vi "HipEXO_SM_BioTorq.vi"(6 "Ext T":dbl, 9 "Trigger Ratio":dbl, 10 "Flex T":dbl, 11 "Hip Angle":dbl) -> (1 "GC Duration":u32, 2 "Extension":bool=TRUE, 3 "Flexion":bool=TRUE, 4 "Output Torque":dbl)   [LabVIEW 2018]
uses:
  <vilib>/functionblocks/Edge Detection/One Shot Rising with Input/One Shot Rising with Input.vi
  <vilib>/functionblocks/FB Core/FB Core.xnode
  <vilib>/functionblocks/NI_FunctionBlock Libraries.lvlib
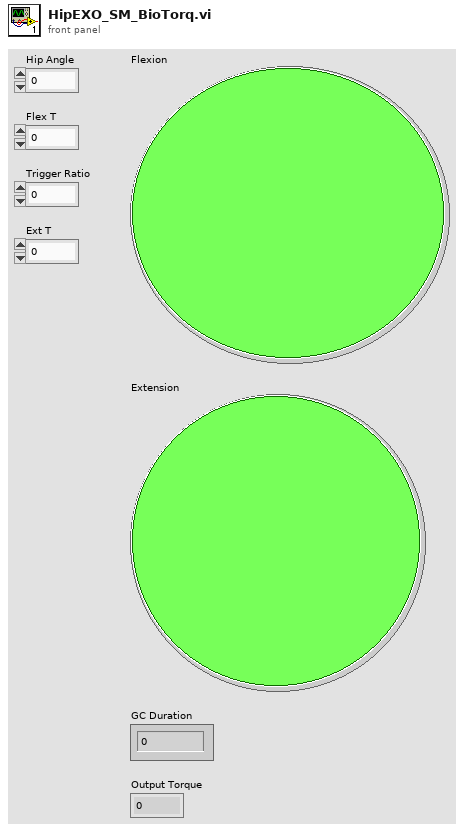
[diagram p1: front panel]
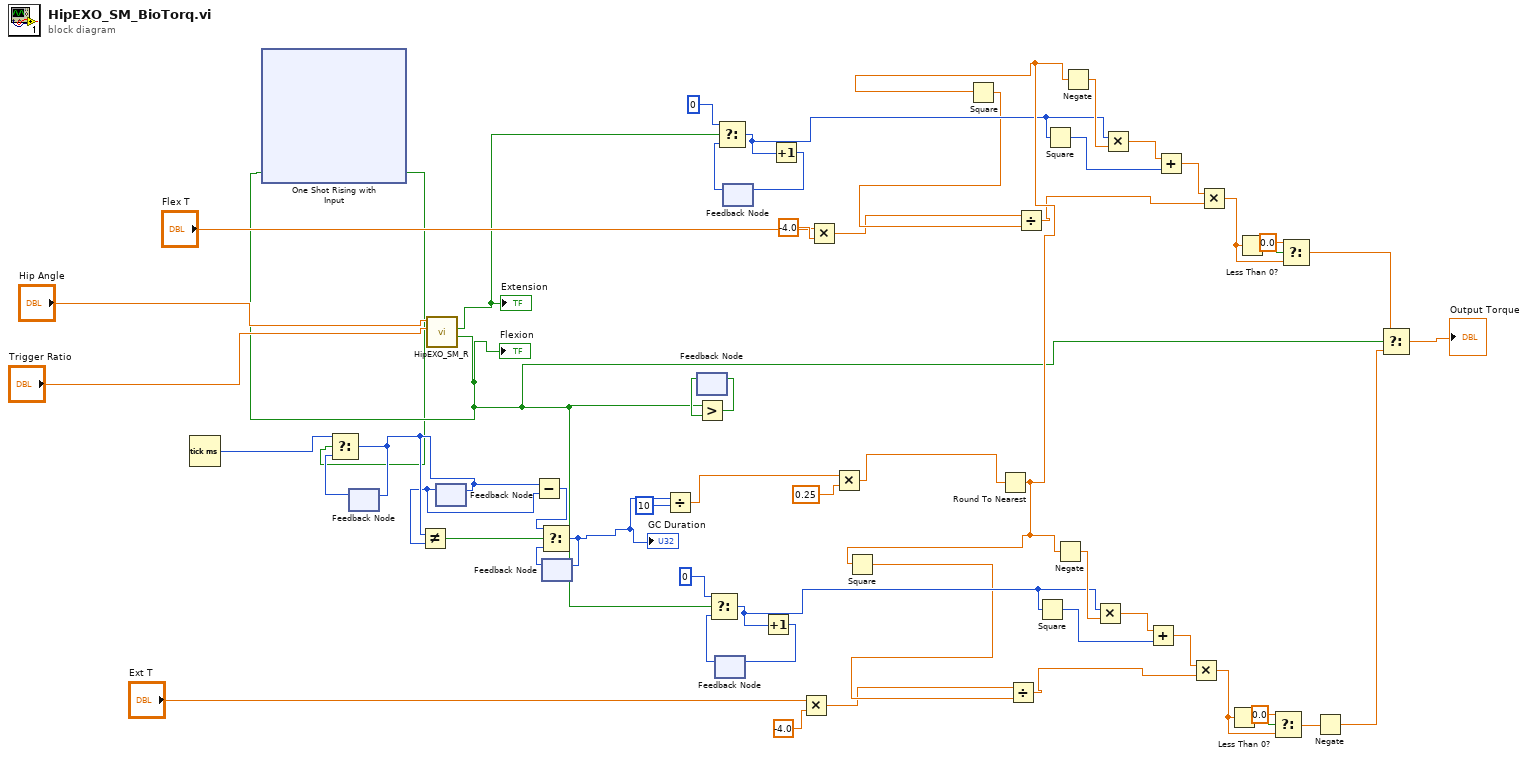
[diagram p0: block diagram]
diagram:
  n1 = Tick Count (ms)() -> (millisecond timer value=w16:u32)
  n2 = feedback #1() -> (w15:u32)  [unwired: 1 in]
  n3 = call "HipEXO_SM_R.vi"("Trigger Ratio"="Trigger Ratio", "Hip Angle"="Hip Angle") -> ("Flexion"=w2:bool, "Extension"=w3:bool)  [unwired: 7 in, 1 out]
  "Extension" <- w3
  "Flexion" <- w2
  n4 = xnode "One Shot Rising with Input"("input"=w2) -> ("output"=w1:bool)  [unwired: 1 in, 1 out]
  n5 = Select(t=w16, s=w1, f=w15) -> (s? t:f=w13:u32)
  n6 = feedback-in #1(w13) -> ()
  n7 = feedback #2() -> (w12:u32)  [unwired: 1 in]
  n8 = Not Equal?(x=w13, y=w12) -> (x != y?=w14:bool)
  n9 = feedback-in #2(w13) -> ()
  n10 = Subtract(x=w13, y=w12) -> (x-y=w11:u32)
  n11 = feedback #3() -> (w10:u32)  [unwired: 1 in]
  n12 = Select(t=w11, s=w14, f=w10) -> (s? t:f=w8:u32)
  "GC Duration" <- w8
  n13 = feedback-in #3(w8) -> ()
  n14 = Divide(x=w8, y=u32 10) -> (x/y=w6:dbl)
  n15 = feedback #4() -> (w17:bool)  [unwired: 1 in]
  n16 = Greater?(x=w2, y=w17) -> (0:w9:bool)
  n17 = feedback-in #4(w9) -> ()
  n18 = feedback #5() -> (w20:u32)  [unwired: 1 in]
  n19 = Select(t=u32 0 ("y"), s=w2, f=w20) -> (s? t:f=w25:u32)
  n20 = feedback #6() -> (w36:u32)  [unwired: 1 in]
  n21 = Select(t=u32 0 ("y"), s=w3, f=w36) -> (s? t:f=w41:u32)
  n22 = Increment(x=w25) -> (x+1=w19:u32)
  n23 = feedback-in #5(w19) -> ()
  n24 = Increment(x=w41) -> (x+1=w35:u32)
  n25 = feedback-in #6(w35) -> ()
  n26 = Multiply(x="Ext T", y=-4.0) -> (x*y=w23:dbl)
  n27 = Multiply(x="Flex T", y=-4.0) -> (x*y=w39:dbl)
  n28 = Multiply(x=w6, y=0.25) -> (x*y=w54:dbl)
  n29 = Round To Nearest(number=w54) -> (nearest integer value=w50:dbl)
  n30 = Square(x=w50) -> (x^2=w24:dbl)
  n31 = Square(x=w50) -> (x^2=w40:dbl)
  n32 = Divide(x=w23, y=w24) -> (x/y=w30:dbl)
  n33 = Divide(x=w39, y=w40) -> (x/y=w46:dbl)
  n34 = Square(x=w25) -> (x^2=w28:u32)
  n35 = Square(x=w41) -> (x^2=w44:u32)
  n36 = Negate(x=w50) -> (-x=w26:dbl)
  n37 = Negate(x=w50) -> (-x=w42:dbl)
  n38 = Multiply(x=w25, y=w26) -> (x*y=w27:dbl)
  n39 = Multiply(x=w41, y=w42) -> (x*y=w43:dbl)
  n40 = Add(x=w27, y=w28) -> (x+y=w29:dbl)
  n41 = Add(x=w43, y=w44) -> (x+y=w45:dbl)
  n42 = Multiply(x=w29, y=w30) -> (x*y=w33:dbl)
  n43 = Multiply(x=w45, y=w46) -> (x*y=w49:dbl)
  n44 = Less Than 0?(x=w33) -> (x < 0?=w31:bool)
  n45 = Less Than 0?(x=w49) -> (x < 0?=w47:bool)
  n46 = Select(t=0.0, s=w31, f=w33) -> (s? t:f=w51:dbl)
  n47 = Select(t=0.0, s=w47, f=w49) -> (s? t:f=w52:dbl)
  n48 = Negate(x=w51) -> (-x=w53:dbl)
  n49 = Select(t=w52, s=w2, f=w53) -> (s? t:f=→"Output Torque":dbl)
